vi "EQ read summary file.vi"(10 "Folder path: equalization reports":path) -> (0 "EQ summary":string, 1 "ID summary":string, 2 "quants px bons per chip":u8[](array[numeric]), 3 "ChipID list":u32[](array[numeric]) format="%.0x")   [LabVIEW 2015, in "VIPM2.lvlib"]
doc: "Llegeix el EQ summary file i construeix les variables per al EQ choose report (EQ report viewer)."
uses:
  VIPM2.lvlib
panel:
  out "Chip data text":string
  out "text from file":string
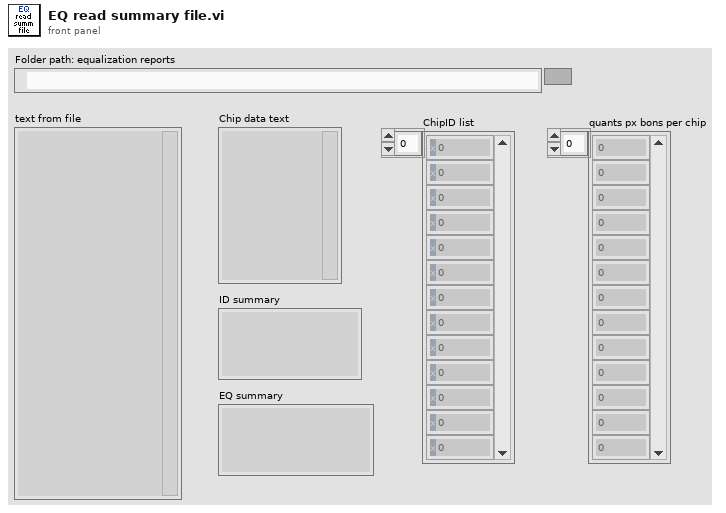
[diagram p1: front panel]
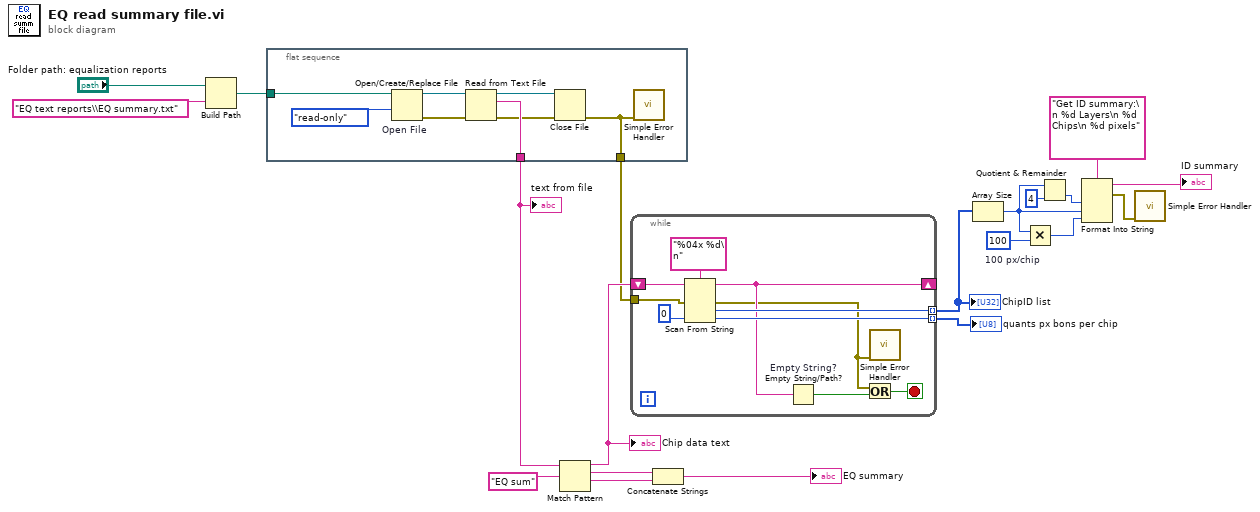
[diagram p0: block diagram]
diagram:
  w8 = 100  # 100 px/chip
  n1 = Build Path(base path="Folder path: equalization reports", name or relative path="EQ text reports\\EQ summary.txt") -> (appended path=w1:path)
  n2 = flat-sequence {
    tunnel: [w27] -> w16
    tunnel: [w22] -> w4
    tunnel: w1 -> [w21]
    frame #0 {
      n3 = Open/Create/Replace File "Open File"(file path (use dialog)=w21, access (0:read/write)=enum16{"read/write", "read-only", "write-only"}."read-only") -> (refnum out=w26:refnum<file>, error out=w25:errorcluster)  [unwired: 4 in, 1 out]
      n4 = Read from Text File(file (use dialog)=w26, error in=w25) -> (refnum out=w24:refnum<file>, text=w27:string, error out=w23:errorcluster)  [unwired: 2 in, 1 out]
      n5 = Close File(refnum=w24, error in=w23) -> (error out=w22:errorcluster)  [unwired: 1 out]
      n6 = call <vilib>:"Simple Error Handler.vi"("error in (no error)"=w22) -> ()  [unwired: 4 in, 5 out]
    }
  }
  n7 = Match Pattern(string=w16, regular expression="EQ sum") -> (before substring=w15:string, match substring=w18:string, after substring=w17:string)  [unwired: 1 in, 1 out]
  "Chip data text" <- w15
  n8 = while {
    shift-right: [w31] -> _
    shift-left: w15 -> [w32]
    tunnel: [w34] -> w12 mode=indexing
    tunnel: [w33] -> w14 mode=indexing
    tunnel: w4 -> [w29]
    stop <- w38 stop-if-true
    n9 = Scan From String "Scan From String"(format string="%04x %d\n", input string=w32, error in=w29, default 2=u8 0 ("default value 2")) -> (remaining string=w31:string, error out=w30:errorcluster, output 1=w34:u32, output 2=w33:u8)  [unwired: 2 in, 1 out]
    n10 = Empty String/Path? "Empty String?"(string/path=w31) -> (empty?=w37:bool)
    n11 = Or(x=w30, y=w37) -> (x .or. y?=w38:bool)
    n12 = call <vilib>:"Simple Error Handler.vi"("error in (no error)"=w30) -> ()  [unwired: 4 in, 5 out]
  }
  "ChipID list" <- w12
  "quants px bons per chip" <- w14
  n13 = Concatenate Strings "Concatenate Strings"(w18, w17) -> (→"EQ summary":string)
  n14 = Array Size(array=w12) -> (size(s)=w9:i32)
  n15 = Multiply(x=w9, y=w8) -> (x*y=w7:i32)
  n16 = Quotient & Remainder(x=w9, y=4) -> (floor(x/y)=w11:i32)  [unwired: 1 out]
  n17 = Format Into String "Format Into String"(format string="Get ID summary:\n %d Layers\n %d Chips\n %d pixels", w11, w9, w7) -> (resulting string=→"ID summary":string, error out=w5:errorcluster)  [unwired: 2 in]
  n18 = call <vilib>:"Simple Error Handler.vi"("error in (no error)"=w5) -> ()  [unwired: 4 in, 5 out]
  "text from file" <- w16
